vi "HFRR ADV v020 new software.vi"() -> ()   [LabVIEW 2025] (continued)
                    n2485 = Concatenate Strings(w3616, w3615, "Fuel Discription :-" ("Substring"), w3626, w3615, w3636, w3615, "Batch Ref Num :-" ("Substring"), w3612, w3615, " Remarks :- " ("Substring"), w3623, w3615, " Date :- " ("Substring"), w3618, w3615, "Tested By :-" ("Substring"), w3620) -> (w3630:string)
                    "REMARKS" <- w3630
                    n2486 = call <vilib>:"Write Characters To File.vi"("append to file? (new file:F)"=FALSE, "character string"=w3632, "file path (dialog if empty)"=w3600) -> ()  [unwired: 2 in, 1 out]
                    n2487 = call <vilib>:"Write Characters To File.vi"("append to file? (new file:F)"=FALSE, "character string"=w3630, "file path (dialog if empty)"=w3599) -> ()  [unwired: 2 in, 1 out]
                  }
                  frame #2 {
                    n2488 = local write "Cycles elapsed"(0 ("Cycles elapsed")) -> ()
                    n2489 = local write "cyclecount"(0 ("cyclecount")) -> ()
                    n2490 = local write "Save & Continue"(FALSE ("OK")) -> ()
                    n2491 = local write "autostrtflg"(TRUE ("autostrtflg")) -> ()
                    n2492 = local write "Save"(FALSE ("Save")) -> ()
                    n2493 = Get Date/Time In Seconds() -> (seconds since 1Jan1904=w3655:timestamp)
                    n2494 = To Double Precision Float(number=w3655) -> (double precision float=w3654:dbl)
                    n2495 = local write "acq timer"(w3654) -> ()
                    n2496 = One Button Dialog(message="Please ensure sample is mounted properly and machine is ready in all aspects for testing !", button name ("OK")="Ok") -> ()  [unwired: 1 out]
                  }
                  frame #3 {
                    n2497 = stacked-sequence {
                      frame #0 {
                        n2498 = local write "Main Dashboard Buttons"(T1."Dashboard" ("Main Dashboard Buttons")) -> ()
                        n2499 = local write "Main Tab"(T2."Acquire" ("Main Tab")) -> ()
                      }
                      frame #1 {
                        n2500 = local write "EVENT LOG"("" ("EVENT LOG")) -> ()
                      }
                      frame #2 {
                        n2501 = Wait (ms)(milliseconds to wait=u32 50) -> ()  [unwired: 1 out]
                      }
                      frame #3 {
                        n2502 = disable-structure shown="Disabled" {
                          frame Disabled {
                            n2503 = local read "EVENT LOG"() -> (w3667:string)
                            n2504 = call "Event Log.vi"("Content"="Test Details", "EVENT LOG"=w3667) -> ("EVENT LOG"=w3666:string)  [unwired: 8 in, 1 out]
                            n2505 = local write "EVENT LOG"(w3666) -> ()
                          }
                          frame Enabled {
                          }
                        }
                      }
                      frame #4 {
                        n2506 = Wait (ms)(milliseconds to wait=u32 50) -> ()  [unwired: 1 out]
                      }
                      frame #5 {
                        n2507 = local read "FILE"() -> (w3669:string)
                        n2508 = Concatenate Strings("File Name :" ("Content"), w3669) -> (w3670:string)
                        n2509 = local read "EVENT LOG"() -> (w3673:string)
                        n2510 = call "Event Log.vi"("Content"=w3670, "EVENT LOG"=w3673) -> ("EVENT LOG"=w3672:string)  [unwired: 8 in, 1 out]
                        n2511 = local write "EVENT LOG"(w3672) -> ()
                      }
                      frame #6 {
                        n2512 = Wait (ms)(milliseconds to wait=u32 50) -> ()  [unwired: 1 out]
                      }
                      frame #7 {
                        n2513 = local read "Batch Ref Num :"() -> (w3675:string)
                        n2514 = Concatenate Strings("Batch Ref No :" ("Content"), w3675) -> (w3676:string)
                        n2515 = local read "EVENT LOG"() -> (w3679:string)
                        n2516 = call "Event Log.vi"("Content"=w3676, "EVENT LOG"=w3679) -> ("EVENT LOG"=w3678:string)  [unwired: 8 in, 1 out]
                        n2517 = local write "EVENT LOG"(w3678) -> ()
                      }
                      frame #8 {
                        n2518 = Wait (ms)(milliseconds to wait=u32 50) -> ()  [unwired: 1 out]
                      }
                      frame #9 {
                        n2519 = local read "tested by"() -> (w3681:string)
                        n2520 = Concatenate Strings("Tested By :" ("Content"), w3681) -> (w3682:string)
                        n2521 = local read "EVENT LOG"() -> (w3685:string)
                        n2522 = call "Event Log.vi"("Content"=w3682, "EVENT LOG"=w3685) -> ("EVENT LOG"=w3684:string)  [unwired: 8 in, 1 out]
                        n2523 = local write "EVENT LOG"(w3684) -> ()
                      }
                      frame #10 {
                        n2524 = Wait (ms)(milliseconds to wait=u32 50) -> ()  [unwired: 1 out]
                      }
                      frame #11 {
                        n2525 = local read "TEST STANDARD"() -> (w3688:T3)
                        n2526 = case shown="\"ASTM D6079\", Default" w3688 {
                          tunnel: ["ASTM D6079" "ISO 12156" "CEC F-096-A-06" "Custom"] -> w3687
                          frame "ASTM D6079", Default {
                          }
                          frame "ISO 12156" {
                          }
                          frame "CEC F-096-A-06" {
                          }
                          frame "Custom" {
                          }
                        }
                        n2527 = Concatenate Strings("Test Standard :" ("Content"), w3687) -> (w3689:string)
                        n2528 = local read "EVENT LOG"() -> (w3692:string)
                        n2529 = call "Event Log.vi"("Content"=w3689, "EVENT LOG"=w3692) -> ("EVENT LOG"=w3691:string)  [unwired: 8 in, 1 out]
                        n2530 = local write "EVENT LOG"(w3691) -> ()
                      }
                      frame #12 {
                        n2531 = Wait (ms)(milliseconds to wait=u32 50) -> ()  [unwired: 1 out]
                      }
                      frame #13 {
                        n2532 = local read "Fuel Discription :"() -> (w3698:string)
                        n2533 = Concatenate Strings("Fuel Description :" ("Content"), w3698) -> (w3699:string)
                        n2534 = local read "EVENT LOG"() -> (w3702:string)
                        n2535 = call "Event Log.vi"("Content"=w3699, "EVENT LOG"=w3702) -> ("EVENT LOG"=w3701:string)  [unwired: 8 in, 1 out]
                        n2536 = local write "EVENT LOG"(w3701) -> ()
                      }
                      frame #14 {
                        n2537 = Wait (ms)(milliseconds to wait=u32 50) -> ()  [unwired: 1 out]
                      }
                      frame #15 {
                        n2538 = local read "Remarks :"() -> (w3704:string)
                        n2539 = Concatenate Strings("Remarks :" ("Content"), w3704) -> (w3705:string)
                        n2540 = local read "EVENT LOG"() -> (w3708:string)
                        n2541 = call "Event Log.vi"("Content"=w3705, "EVENT LOG"=w3708) -> ("EVENT LOG"=w3707:string)  [unwired: 8 in, 1 out]
                        n2542 = local write "EVENT LOG"(w3707) -> ()
                      }
                      frame #16 {
                        n2543 = Wait (ms)(milliseconds to wait=u32 50) -> ()  [unwired: 1 out]
                      }
                      frame #17 {
                        n2544 = local read "Operator ID"() -> (w3710:string)
                        n2545 = Concatenate Strings("Operator ID :" ("Content"), w3710) -> (w3712:string)
                        n2546 = local read "EVENT LOG"() -> (w3714:string)
                        n2547 = call "Event Log.vi"("Content"=w3712, "EVENT LOG"=w3714) -> ("EVENT LOG"=w3713:string)  [unwired: 8 in, 1 out]
                        n2548 = local write "EVENT LOG"(w3713) -> ()
                      }
                      frame #18 {
                        n2549 = Wait (ms)(milliseconds to wait=u32 50) -> ()  [unwired: 1 out]
                      }
                      frame #19 {
                        n2550 = disable-structure shown="Disabled" {
                          frame Disabled {
                            n2551 = local read "EVENT LOG"() -> (w3718:string)
                            n2552 = call "Event Log.vi"("Content"="Test Parameter", "EVENT LOG"=w3718) -> ("EVENT LOG"=w3717:string)  [unwired: 8 in, 1 out]
                            n2553 = local write "EVENT LOG"(w3717) -> ()
                          }
                          frame Enabled {
                          }
                        }
                      }
                      frame #20 {
                        n2554 = Wait (ms)(milliseconds to wait=u32 50) -> ()  [unwired: 1 out]
                      }
                      frame #21 {
                        n2555 = local read "Set Hz"() -> (w3722:dbl)
                        n2556 = Number To Fractional String(number=w3722, precision (6)=i16 2) -> (F-format string=w3721:string)  [unwired: 2 in]
                        n2557 = Concatenate Strings("Set Frequency [Hz] :" ("Content"), w3721) -> (w3724:string)
                        n2558 = local read "EVENT LOG"() -> (w3726:string)
                        n2559 = call "Event Log.vi"("Content"=w3724, "EVENT LOG"=w3726) -> ("EVENT LOG"=w3725:string)  [unwired: 8 in, 1 out]
                        n2560 = local write "EVENT LOG"(w3725) -> ()
                      }
                      frame #22 {
                        n2561 = Wait (ms)(milliseconds to wait=u32 50) -> ()  [unwired: 1 out]
                      }
                      frame #23 {
                        n2562 = local read "NORMAL LOAD"() -> (w3729:dbl)
                        n2563 = Number To Fractional String(number=w3729, precision (6)=i16 2) -> (F-format string=w3730:string)  [unwired: 2 in]
                        n2564 = Concatenate Strings("Applied Load [grams] :" ("Content"), w3730) -> (w3732:string)
                        n2565 = local read "EVENT LOG"() -> (w3734:string)
                        n2566 = call "Event Log.vi"("Content"=w3732, "EVENT LOG"=w3734) -> ("EVENT LOG"=w3733:string)  [unwired: 8 in, 1 out]
                        n2567 = local write "EVENT LOG"(w3733) -> ()
                      }
                      frame #24 {
                        n2568 = Wait (ms)(milliseconds to wait=u32 50) -> ()  [unwired: 1 out]
                      }
                      frame #25 {
                        n2569 = local read "Set Strk"() -> (w3737:dbl)
                        n2570 = Number To Fractional String(number=w3737, precision (6)=i16 2) -> (F-format string=w3738:string)  [unwired: 2 in]
                        n2571 = Concatenate Strings("Set Stroke [mm] :" ("Content"), w3738) -> (w3740:string)
                        n2572 = local read "EVENT LOG"() -> (w3742:string)
                        n2573 = call "Event Log.vi"("Content"=w3740, "EVENT LOG"=w3742) -> ("EVENT LOG"=w3741:string)  [unwired: 8 in, 1 out]
                        n2574 = local write "EVENT LOG"(w3741) -> ()
                      }
                      frame #26 {
                        n2575 = Wait (ms)(milliseconds to wait=u32 50) -> ()  [unwired: 1 out]
                      }
                      frame #27 {
                        n2576 = local read "Set Temp"() -> (w3745:dbl)
                        n2577 = Number To Fractional String(number=w3745, precision (6)=i16 2) -> (F-format string=w3746:string)  [unwired: 2 in]
                        n2578 = Concatenate Strings("Set Temperature [deg C] :" ("Content"), w3746) -> (w3748:string)
                        n2579 = local read "EVENT LOG"() -> (w3750:string)
                        n2580 = call "Event Log.vi"("Content"=w3748, "EVENT LOG"=w3750) -> ("EVENT LOG"=w3749:string)  [unwired: 8 in, 1 out]
                        n2581 = local write "EVENT LOG"(w3749) -> ()
                      }
                      frame #28 {
                        n2582 = Wait (ms)(milliseconds to wait=u32 50) -> ()  [unwired: 1 out]
                      }
                      frame #29 {
                        n2583 = local read "Set Rh"() -> (w3753:dbl)
                        n2584 = Number To Fractional String(number=w3753, precision (6)=i16 2) -> (F-format string=w3754:string)  [unwired: 2 in]
                        n2585 = Concatenate Strings("Set Humidity [%RH] :" ("Content"), w3754) -> (w3756:string)
                        n2586 = local read "EVENT LOG"() -> (w3758:string)
                        n2587 = call "Event Log.vi"("Content"=w3756, "EVENT LOG"=w3758) -> ("EVENT LOG"=w3757:string)  [unwired: 8 in, 1 out]
                        n2588 = local write "EVENT LOG"(w3757) -> ()
                      }
                      frame #30 {
                        n2589 = Wait (ms)(milliseconds to wait=u32 50) -> ()  [unwired: 1 out]
                      }
                      frame #31 {
                        n2590 = local read "test time"() -> (w3761:dbl)
                        n2591 = Number To Fractional String(number=w3761, precision (6)=i16 1) -> (F-format string=w3762:string)  [unwired: 2 in]
                        n2592 = Concatenate Strings("Test Duration [mins] :" ("Content"), w3762) -> (w3764:string)
                        n2593 = local read "EVENT LOG"() -> (w3766:string)
                        n2594 = call "Event Log.vi"("Content"=w3764, "EVENT LOG"=w3766) -> ("EVENT LOG"=w3765:string)  [unwired: 8 in, 1 out]
                        n2595 = local write "EVENT LOG"(w3765) -> ()
                      }
                      frame #32 {
                        w3767 = dbl[] [] ("History Data")
                        w3768 = cluster{"y":dbl, dbl, "y":dbl}[] [] ("History Data")
                        w3769 = FALSE ("Visible")
                        n2596 = property on="Stroke ( mm )" class="WFChart (strict)"("History Data"=w3768) -> ()  [unwired: 2 in, 2 out]
                        n2597 = property on="Humidity ( %RH )" class="WFChart (strict)"("History Data"=w3767) -> ()  [unwired: 2 in, 2 out]
                        n2598 = property on="Temperature ( Deg C )" class="WFChart (strict)"("History Data"=w3767) -> ()  [unwired: 2 in, 2 out]
                        n2599 = property on="Electrical Contact Resistance ( % )" class="WFChart (strict)"("History Data"=w3767) -> ()  [unwired: 2 in, 2 out]
                        n2600 = property on="Coefficient of Friction" class="WFChart (strict)"("History Data"=w3767) -> ()  [unwired: 2 in, 2 out]
                        n2601 = property on="Frictional Force ( N )" class="WFChart (strict)"("History Data"=w3767) -> ()  [unwired: 2 in, 2 out]
                        n2602 = property on="Coefficient of Friction" class="WFChart (strict)"("History Data"=w3767) -> ()  [unwired: 2 in, 2 out]
                        n2603 = property on="Frictional Force ( N )" class="WFChart (strict)"("History Data"=w3767) -> ()  [unwired: 2 in, 2 out]
                        n2604 = property on="Electrical Contact Resistance ( % )" class="WFChart (strict)"("History Data"=w3767) -> ()  [unwired: 2 in, 2 out]
                        n2605 = property on="Humidity ( %RH )" class="WFChart (strict)"("History Data"=w3767) -> ()  [unwired: 2 in, 2 out]
                        n2606 = property on="Stroke ( mm )" class="WFChart (strict)"("History Data"=w3768) -> ()  [unwired: 2 in, 2 out]
                        n2607 = property on="Temperature ( Deg C )" class="WFChart (strict)"("History Data"=w3767) -> ()  [unwired: 2 in, 2 out]
                        n2608 = property on="Service Password Log" class="Str"("Visible"=w3769) -> ()  [unwired: 2 in, 2 out]
                        n2609 = property on="Password 3" class="Clust (strict)"("Visible"=w3769) -> ()  [unwired: 2 in, 2 out]
                      }
                    }
                    "TEST FILE NAM,E SAVED" <- TRUE ("TEST FILE NAM,E SAVED")
                  }
                }
              }
            }
          }
        }
        n2610 = case shown="True" w3066 {
          frame False {
            n2611 = local write "tfalg"(0.0 ("tfalg")) -> ()
          }
          frame True {
            n2612 = local read "tfalg"() -> (w3211:dbl)
            n2613 = Equal?(x=w3211, y=0.0) -> (x = y?=w3212:bool)
            n2614 = case shown="True" w3212 {
              frame False {
              }
              frame True {
                n2615 = local read "Total No. of Tests"() -> (w3215:dbl)
                n2616 = local write "tfalg"(1.0 ("tfalg")) -> ()
                n2617 = local write "acq 2"(FALSE ("acq 2")) -> ()
                n2618 = Wait (ms)(milliseconds to wait=u32 200) -> ()  [unwired: 1 out]
                n2619 = Increment(x=w3215) -> (x+1=w3214:dbl)
                n2620 = local write "Total No. of Tests"(w3214) -> ()
              }
            }
          }
        }
        n2621 = local write "Test \nStatus"(w3072) -> ()
        n2622 = local write "Save"(w3072) -> ()
        n2623 = local read "Main Tab"() -> (w3029:T2)
        n2624 = case shown="True" w3053 {
          tunnel: [FALSE ("RUN") TRUE ("RUN")] -> w3052
          tunnel: [_ 1] -> w3045
          frame False {
          }
          frame True {
          }
        }
        n2625 = In Range and Coerce(upper limit=w3060, x=w3033, lower limit=w3059) -> (In Range?=w3051:bool)  [unwired: 1 out]
        n2626 = In Range and Coerce(upper limit=w3057, x=w3032, lower limit=w3058) -> (In Range?=w3049:bool)  [unwired: 1 out]
        n2627 = case shown="True" w3065 {
          frame False {
            n2628 = local read "Rt 3"() -> (w3193:bool)
            n2629 = case shown="True" w3193 {
              frame False {
              }
              frame True {
                n2630 = local write "Rt 3"(FALSE ("Rt 3")) -> ()
                n2631 = local write "Json End Flg"(TRUE ("Upld AR 2")) -> ()
              }
            }
            "Rt" <- TRUE ("Rt")
            "Rt 2" <- FALSE ("Rt")
          }
          frame True {
            n2632 = local read "Rt"() -> (w3200:bool)
            n2633 = local write "Rt 2"(TRUE ("Rt 2")) -> ()
            n2634 = case shown="True" w3200 {
              frame False {
              }
              frame True {
                w3201 = TRUE ("Upld AR 2")
                n2635 = local write "Rt"(FALSE ("Rt")) -> ()
                n2636 = local write "Upld AR"(w3201) -> ()
                n2637 = local write "Json St Flg"(w3201) -> ()
              }
            }
            "Rt 3" <- TRUE ("Rt 3")
          }
        }
        n2638 = case shown="True" w3051 {
          tunnel: [FALSE ("RUN") TRUE ("RUN")] -> w3050
          tunnel: [_ 2] -> w3044
          frame False {
          }
          frame True {
          }
        }
        n2639 = case shown="True" w3049 {
          tunnel: [FALSE ("RUN") TRUE ("RUN")] -> w3048
          tunnel: [_ 3] -> w3043
          frame False {
          }
          frame True {
          }
        }
        n2640 = case shown="\"Acquire\"" w3029 {
          tunnel: w3031 -> [_ w3262]
          frame Default {
            w3261 = 0.0 ("output")
            n2641 = local write "PID-out"(w3261) -> ()
            n2642 = local write "Frequency ( Hz )"(w3261) -> ()
          }
          frame "Acquire" {
            n2643 = stacked-sequence {
              frame #0 {
                n2644 = local read "Auto Start Test"() -> (w3264:bool)
                n2645 = case shown="True" w3264 {
                  tunnel: "RUN" -> [w3285 w3288]
                  tunnel: [w3285 w3287] -> w3265
                  frame False {
                  }
                  frame True {
                    n2646 = local read "Auto Start Temp"() -> (w3286:bool)
                    n2647 = Or(x=w3288, y=w3286) -> (x .or. y?=w3287:bool)
                  }
                }
                n2648 = local read "clk"() -> (w3284:dbl)
                n2649 = local read "Save"() -> (w3280:bool)
                n2650 = Equal?(x=w3284, y=0.0) -> (x = y?=w3281:bool)
                n2651 = And(x=w3281, y=w3280) -> (x .and. y?=w3282:bool)
                n2652 = Not(x="Engage") -> (.not. x?=w3271:bool)
                n2653 = case shown="False" w3265 {
                  tunnel: [0.0 w3311] -> w3267
                  frame False {
                    (unwired) TRUE ("Visible")
                    n2654 = local read "Auto Start Test"() -> (w3292:bool)
                    n2655 = local write "Start Time"(TRUE ("Start Time")) -> ()
                    n2656 = property on="Stroke 2" class="DigNum (strict)"("Visible"=FALSE) -> ()  [unwired: 2 in, 2 out]
                    n2657 = case shown="False" w3292 {
                      frame False {
                        n2658 = property on="Heater Button" class="Bool (strict)"("DisabledEnum"=T19."Enabled" ("Disabled")) -> ()  [unwired: 2 in, 2 out]
                        n2659 = property on="Humidity" class="Bool (strict)"("DisabledEnum"=T19."Enabled" ("Disabled")) -> ()  [unwired: 2 in, 2 out]
                      }
                      frame True {
                      }
                    }
                    n2660 = case shown="False" "TestCompFlg" {
                      frame False {
                        n2661 = local read "StartFlg"() -> (w3300:bool)
                        n2662 = case shown="True" w3300 {
                          frame False {
                          }
                          frame True {
                            n2663 = stacked-sequence {
                              frame #0 {
                                n2664 = local read "EVENT LOG"() -> (w3304:string)
                                n2665 = call "Event Log.vi"("Content"="Test was interrupted", "EVENT LOG"=w3304) -> ("EVENT LOG"=w3305:string)  [unwired: 8 in, 1 out]
                                n2666 = local write "EVENT LOG"(w3305) -> ()
                                n2667 = property on="RUN" class="Bool (strict)"("Visible"=TRUE) -> ()  [unwired: 2 in, 2 out]
                                n2668 = property on="Auto Start Test" class="Bool (strict)"("Visible"=TRUE) -> ()  [unwired: 2 in, 2 out]
                              }
                              frame #1 {
                                w3307 = FALSE ("StartFlg")
                                n2669 = property on="Heater Button" class="Bool (strict)"("Val(Sgnl)"=FALSE ("Value (Signaling)")) -> ()  [unwired: 2 in, 2 out]
                                n2670 = local write "Heater Button"(w3307) -> ()
                                n2671 = local write "StartFlg"(w3307) -> ()
                                n2672 = local write "Humidity"(w3307) -> ()
                              }
                              frame #2 {
                                n2673 = local write "Command"("VC;0" ("Command")) -> ()
                              }
                              frame #3 {
                                n2674 = Wait (ms)(milliseconds to wait=u32 1500) -> ()  [unwired: 1 out]
                              }
                              frame #4 {
                                n2675 = local write "Command"("HE;0" ("Command")) -> ()
                              }
                            }
                          }
                        }
                      }
                      frame True {
                      }
                    }
                    n2676 = local write "String 14"("Test will autostart once parameters reach the set value." ("String 14")) -> ()
                  }
                  frame True {
                    (unwired) FALSE ("Visible")
                    n2677 = property on="Stroke 2" class="DigNum (strict)"("Visible"=TRUE) -> ()  [unwired: 2 in, 2 out]
                    n2678 = property on="STOP 2" class="Bool (strict)"("Disabled"=u8 2) -> ()  [unwired: 2 in, 2 out]
                    n2679 = local write "String 14"(" Running....." ("String 14")) -> ()
                    n2680 = property on="Heater Button" class="Bool (strict)"("DisabledEnum"=T19."Disabled and Grayed Out" ("Disabled")) -> ()  [unwired: 2 in, 2 out]
                    n2681 = property on="Humidity" class="Bool (strict)"("DisabledEnum"=T19."Disabled and Grayed Out" ("Disabled")) -> ()  [unwired: 2 in, 2 out]
                    n2682 = case shown="True" "Start Time" {
                      selector: "Start Time" -> [_ w3330]
                      frame False {
                      }
                      frame True {
                        n2683 = Not(x=w3330) -> (.not. x?=w3329:bool)
                        n2684 = local write "Start Time"(w3329) -> ()
                        n2685 = local read "EVENT LOG"() -> (w3331:string)
                        n2686 = call "Event Log.vi"("Content"="Test in progress", "EVENT LOG"=w3331) -> ("EVENT LOG"=w3333:string)  [unwired: 8 in, 1 out]
                        n2687 = local write "EVENT LOG"(w3333) -> ()
                      }
                    }
                    n2688 = disable-structure shown="Enabled" {
                      disable-tunnel: [w3322 w3328] -> w3311
                      frame Disabled {
                        n2689 = local read "Set Hz"() -> (w3325:dbl)
                        n2690 = call <vilib>:"Uniform White Noise Waveform.vi"() -> ("signal out"=w3324:waveform(dbl))  [unwired: 10 in, 1 out]
                        n2691 = Random Number (0-1)() -> (number: 0 to 1=w3321:dbl)
                        n2692 = Add(x=w3325, y=w3324) -> (x+y=w3323:waveform(dbl))
                        n2693 = Multiply(x=ext 0.01 ("y"), y=w3321) -> (x*y=w3319:ext)
                        n2694 = Multiply(x=w3323, y=w3319) -> (x*y=w3322:waveform(ext))
                      }
                      frame Enabled {
                        n2695 = call-poly <vilib>:"Random Number (Range).vi"("lower bound (0)"=49.89, "upper bound (100)"=50.8) -> ("number"=w3328:dbl)  [unwired: 9 in]
                      }
                    }
                    "StartFlg" <- TRUE ("StartFlg")
                  }
                }
                n2696 = case shown="True" w3282 {
                  frame False {
                  }
                  frame True {
                    n2697 = local write "clk"(10.0 ("clk")) -> ()
                    n2698 = Get Date/Time In Seconds() -> (seconds since 1Jan1904=w3336:timestamp)
                    n2699 = To Double Precision Float(number=w3336) -> (double precision float=w3334:dbl)
                    n2700 = local write "acq timer"(w3334) -> ()
                    n2701 = local write "act save time"(w3334) -> ()
                  }
                }
                n2702 = call "Elapsed Time"("Time Target (s)"="Countdown", "Reset"=w3271) -> ("Elapsed Time (s)"=w3276:dbl, "Time has Elapsed"=w3274:bool)  [unwired: 10 in, 6 out]
                "Countdown 2" <- w3276
                n2703 = Subtract(x=w3276, y=2.0) -> (x-y=w3279:dbl)
                n2704 = Less?(x=w3279, y="Countdown") -> (x < y?=w3277:bool)
                n2705 = And(x=w3277, y=w3274) -> (x .and. y?=w3273:bool)
                n2706 = case shown="True" w3273 {
                  frame False {
                  }
                  frame True {
                    (unwired) dbl[] [] ("History Data")
                    n2707 = local write "Engage"(FALSE ("Engage")) -> ()
                    n2708 = local write "RUN"(TRUE ("RUN")) -> ()
                    n2709 = local read "Humidity ( %RH )"() -> (→"Rh Before":dbl)
                  }
                }
                n2710 = local read "Test \nStatus"() -> (w3269:bool)
                n2711 = Select(t=w3267, s=w3269, f=0.0) -> (s? t:f=w3268:dbl)
                n2712 = local write "Frequency ( Hz )"(w3268) -> ()
              }
              frame #1 {
                w3359 = 1000000.0 ("x")
                # "HC;1/0\nST;VALUE"
                # "Elapsed time\ncof\nstroke\nAir temp\nTemp\nHumidity"
                # "acq timer\n\nact save time"
                # "convert to microseconds"
                n2713 = local read "COUNT"() -> (w3342:i32)
                n2714 = local read "Rate"() -> (w3355:dbl)
                n2715 = Divide(x=w3359, y=w3355) -> (x/y=w3360:dbl)
                n2716 = Greater Or Equal?(x=w3342, y=250) -> (x >= y?=w3341:bool)
                n2717 = Get Date/Time In Seconds() -> (seconds since 1Jan1904=w3362:timestamp)
                n2718 = case shown="True" w3341 {
                  frame False {
                    n2719 = local read "COUNT"() -> (w3363:i32)
                    n2720 = Increment(x=w3363) -> (x+1=w3364:i32)
                    n2721 = local write "COUNT"(w3364) -> ()
                  }
                  frame True {
                    n2722 = local write "COUNT"(0 ("COUNT")) -> ()
                  }
                }
                n2723 = local read "Samplingtime 2"() -> (w3340:dbl)
                n2724 = local read "act save time"() -> (w3357:dbl)
                n2725 = Divide(x=w3360, y=w3359) -> (x/y=w3358:dbl)
                n2726 = To Double Precision Float(number=w3362) -> (double precision float=w3351:dbl)
                n2727 = Add(x=w3357, y=w3340) -> (x+y=w3356:dbl)
                n2728 = local read "acq timer"() -> (w3361:dbl)
                n2729 = local read "COUNT"() -> (w3344:i32)
                n2730 = Greater Or Equal?(x=w3351, y=w3356) -> (x >= y?=w3339:bool)
                n2731 = Multiply(x=w3358, y=w3344) -> (x*y=w3350:dbl)
                n2732 = Subtract(x=w3351, y=w3361) -> (x-y=w3353:dbl)
                n2733 = local read "Save"() -> (w3354:bool)
                n2734 = Add(x=w3353, y=w3350) -> (x+y=w3337:dbl)
                "Elapsed time 3" <- w3337
                n2735 = And(x=w3339, y=w3354) -> (x .and. y?=w3352:bool)
                n2736 = Divide(x=w3337, y=60.0) -> (x/y=w3348:dbl)
                n2737 = local read "Test \nStatus"() -> (w3338:bool)
                n2738 = local read "clk"() -> (w3345:dbl)
                n2739 = Equal?(x=w3345, y=10.0) -> (x = y?=w3347:bool)
                n2740 = case shown="True" w3352 {
                  tunnel: w3351 -> [_ w3475]
                  tunnel: [FALSE ("Boolean 2") TRUE ("Boolean 2")] -> _
                  frame False {
                  }
                  frame True {
                    w3429 = ";" ("Substring")
                    # "Pid out/\nFreq response value"
                    n2741 = local write "act save time"(w3475) -> ()
                    n2742 = local read "FILE"() -> (w3423:string)
                    n2743 = call "file check.vi"("file name in"=w3423) -> ("error out"=w3426:errorcluster, "file name out"=w3421:string)  [unwired: 9 in]
                    n2744 = local read "LVDT STROKE"() -> (w3418:dbl)
                    n2745 = local read "Add up Stroke"() -> (w3416:dbl)
                    n2746 = call "FILE PATH CREATION.vi"("error in"=w3426, "FILE NAME :"=w3421) -> ("FILE OUT"=w3424:path)  [unwired: 8 in, 1 out]
                    n2747 = Concatenate Strings(w3421, ".dgf" ("Substring")) -> (w3425:string)
                    n2748 = Subtract(x=w3418, y=w3416) -> (x-y=w3417:dbl)
                    n2749 = Absolute Value(x=w3417) -> (abs(x)=w3415:dbl)
                    n2750 = local read "FF 2"() -> (→"Frictional Force ( N )" →"Frictional Force ( N )":dbl)
                    n2751 = Build Path(base path=w3424, name or relative path=w3425) -> (appended path=w3420:path)
                    n2752 = local read "COF 2"() -> (w3434:dbl)
                    "cof" <- w3434
                    "Coefficient of Friction" <- w3434
                    "COF 4" <- w3434
                    "Coefficient of Friction" <- w3434
                    n2753 = local read "TEMP"() -> (w3437:dbl)
                    "Temp" <- w3437
                    "Temperature ( Deg C )" <- w3437
                    n2754 = local read "Humidity ( %RH )"() -> (w3436:dbl)
                    "Humidity ( %RH )" <- w3436
                    "Humidity ( %RH )" <- w3436
                    n2755 = local read "Frequency ( Hz )"() -> (w3443:dbl)
                    n2756 = call <vilib>:"Mean PtByPt.vi"("x"=w3415, "sample length"="STROKE FILTER") -> ("mean"=w3414:dbl)  [unwired: 2 in, 1 out]
                    n2757 = local read "Elapsed time"() -> (w3468:dbl)
                    n2758 = local read "AIR TEMP"() -> (w3441:dbl)
                    n2759 = local read "PID-out"() -> (w3446:dbl)
                    n2760 = local write "Temperature ( Deg C )"(w3437) -> ()
                    n2761 = Number To Fractional String(number=w3414, width (-)=i16 9 ("precision (6)"), precision (6)=i16 6) -> (F-format string=w3461:string)  [unwired: 1 in]
                    n2762 = Number To Fractional String(number=w3441, width (-)=i16 9 ("precision (6)"), precision (6)=i16 3) -> (F-format string=w3460:string)  [unwired: 1 in]
                    n2763 = Number To Fractional String(number=w3437, width (-)=i16 9 ("precision (6)"), precision (6)=i16 3) -> (F-format string=w3457:string)  [unwired: 1 in]
                    n2764 = Number To Fractional String(number=w3436, width (-)=i16 9 ("precision (6)"), precision (6)=i16 3) -> (F-format string=w3454:string)  [unwired: 1 in]
                    n2765 = Number To Fractional String(number=0.0, width (-)=i16 9 ("precision (6)"), precision (6)=i16 3) -> (F-format string=w3451:string)  [unwired: 1 in]
                    n2766 = Number To Fractional String(number=w3446, width (-)=i16 9 ("precision (6)"), precision (6)=i16 3) -> (F-format string=w3447:string)  [unwired: 1 in]
                    n2767 = Number To Fractional String(number=w3443, width (-)=i16 9 ("precision (6)"), precision (6)=i16 3) -> (F-format string=w3442:string)  [unwired: 1 in]
                    n2768 = Number To Fractional String(number=w3434, width (-)=i16 9 ("precision (6)"), precision (6)=i16 6) -> (F-format string=w3469:string)  [unwired: 1 in]
                    n2769 = Number To Fractional String(number=w3468, width (-)=i16 14 ("precision (6)"), precision (6)=i16 3) -> (F-format string=w3470:string)  [unwired: 1 in]
                    n2770 = Bundle("y"=1.02, "mean"=w3414, "y"=0.98) -> (w3435:cluster{"y":dbl, "mean":dbl, "y":dbl})  [unwired: 1 in]
                    n2771 = Number To Fractional String(number="Ambient Humidity :", width (-)=i16 9 ("precision (6)"), precision (6)=i16 6) -> (F-format string=w3427:string)  [unwired: 1 in]
                    n2772 = local read "RUN"() -> (w3433:bool)
                    n2773 = case shown="True" w3433 {
                      tunnel: w3435 -> [_ w3480]
                      tunnel: w3414 -> [_ w3479]
                      tunnel: w3414 -> [_ w3477]
                      tunnel: w3414 -> [_ w3478]
                      frame False {
                      }
                      frame True {
                        "Stroke ( mm )" <- w3480
                        "Stroke ( mm )" <- w3480
                        "Stroke 4" <- w3479
                        "Stroke 3" <- w3477
                        "Stroke 2" <- w3478
                        "measured_stroke" <- w3477
                      }
                    }
                    n2774 = Concatenate Strings(w3470, w3429, w3469, w3429, w3461, w3429, w3460, w3429, w3457, w3429, w3454, w3429, w3451, w3429, w3447, w3429, w3442, w3429, w3427, "\r") -> (w3467:string)
                    n2775 = call <vilib>:"Write Characters To File.vi"("append to file? (new file:F)"=TRUE, "character string"=w3467, "file path (dialog if empty)"=w3420) -> ()  [unwired: 2 in, 1 out]
                    "refresh flag" <- TRUE ("refresh flag")
                  }
                }
                n2776 = case shown="True" w3338 {
                  tunnel: w3348 -> [_ w3374]
                  tunnel: w3353 -> [_ w3384]
                  tunnel: [0.0 w3380] -> _
                  tunnel: w3347 -> [_ w3379]
                  tunnel: [0.0 w3378] -> _
                  tunnel: w3337 -> [_ w3378]
                  tunnel: w3351 -> [w3367 _]
                  frame False {
                    n2777 = local write "acq timer"(w3367) -> ()
                    n2778 = local write "Test Duration Status"(0.0 ("Test Duration Status")) -> ()
                  }
                  frame True {
                    n2779 = local read "Set Hz"() -> (w3381:dbl)
                    n2780 = local write "Elapsed time"(w3374) -> ()
                    n2781 = local read "test time"() -> (w3373:dbl)
                    n2782 = Multiply(x=w3384, y=w3381) -> (x*y=w3383:dbl)
                    n2783 = case shown="False" w3379 {
                      tunnel: w3383 -> [w3385 _]
                      tunnel: [w3385 1.0] -> w3380
                      frame False {
                        n2784 = local write "Cycles elapsed"(w3385) -> ()
                      }
                      frame True {
                      }
                    }
                    n2785 = Greater?(x=w3374, y=w3373) -> (0:w3382:bool)
                    n2786 = Subtract(x=w3373, y=w3374) -> (x-y=w3372:dbl)
                    "time" <- w3372
                    n2787 = Multiply(x=w3372, y=60.0) -> (x*y=w3371:dbl)
                    n2788 = local write "Time Remaining"(w3371) -> ()
                    n2789 = local write "Remaining Time"(w3371) -> ()
                    n2790 = case shown="True" w3382 {
                      frame False {
                      }
                      frame True {
                        n2791 = stacked-sequence {
                          frame #0 {
                            w3390 = T19."Enabled" ("Disabled")
                            w3389 = FALSE ("TEST FILE NAM,E SAVED")
                            w3391 = "" ("FILE")
                            w3392 = TRUE ("Visible")
                            n2792 = local write "Humidity"(FALSE ("Humidity")) -> ()
                            n2793 = local write "RUN"(FALSE ("OK Button 2")) -> ()
                            n2794 = local write "Heater Button"(FALSE ("Heater Button")) -> ()
                            n2795 = local write "Auto Start Test"(FALSE ("Auto Start Test")) -> ()
                            n2796 = local write "TestCompFlg"(TRUE ("StpFlg")) -> ()
                            n2797 = local read "Humidity ( %RH )"() -> (→"Rh After":dbl)
                            n2798 = property on="STOP 2" class="Bool (strict)"("Disabled"=u8 0) -> ()  [unwired: 2 in, 2 out]
                            n2799 = local read "EVENT LOG"() -> (w3397:string)
                            n2800 = call "Event Log.vi"("Content"="Test Completed", "EVENT LOG"=w3397) -> ("EVENT LOG"=w3396:string)  [unwired: 8 in, 1 out]
                            n2801 = property on="RUN" class="Bool (strict)"("Visible"=w3392) -> ()  [unwired: 2 in, 2 out]
                            n2802 = property on="Auto Start Test" class="Bool (strict)"("Visible"=w3392) -> ()  [unwired: 2 in, 2 out]
                            n2803 = local write "Batch Ref Num :"(w3391) -> ()
                            n2804 = local write "FILE"(w3391) -> ()
                            n2805 = local write "EVENT LOG"(w3396) -> ()
                            n2806 = local write "TEST FILE NAM,E SAVED"(w3389) -> ()
                            n2807 = local write "Fuel Discription :"(w3391) -> ()
                            n2808 = local write "START TEMP"(w3389) -> ()
                            n2809 = local write "Remarks :"(w3391) -> ()
                            n2810 = local write "Main Dashboard Buttons"(T1."Imaging" ("Main Dashboard Buttons")) -> ()
                            n2811 = local write "Main Tab"(T2."Adv Scar" ("Main Tab")) -> ()
                            n2812 = property on="FRICVALZ 2" class="Bool (strict)"("DisabledEnum"=w3390) -> ()  [unwired: 2 in, 2 out]
                            n2813 = property on="FRICVALZ 3" class="Bool (strict)"("DisabledEnum"=w3390) -> ()  [unwired: 2 in, 2 out]
                            n2814 = property on="FRICVALZ 4" class="Bool (strict)"("DisabledEnum"=w3390) -> ()  [unwired: 2 in, 2 out]
                          }
                          frame #1 {
                            n2815 = Wait (ms)(milliseconds to wait=u32 1500) -> ()  [unwired: 1 out]
                          }
                          frame #2 {
                            n2816 = local write "Command"("VC;0") -> ()
                          }
                          frame #3 {
                            n2817 = Wait (ms)(milliseconds to wait=u32 1500) -> ()  [unwired: 1 out]
                          }
                          frame #4 {
                            n2818 = local write "Command"("VC;0") -> ()
                          }
                          frame #5 {
                            n2819 = Wait (ms)(milliseconds to wait=u32 1500) -> ()  [unwired: 1 out]
                          }
                          frame #6 {
                            n2820 = local write "Command"("ST;0") -> ()
                          }
                          frame #7 {
                            n2821 = local write "measured_stroke"(0.0 ("measured_stroke")) -> ()
                            n2822 = Wait (ms)(milliseconds to wait=u32 1500) -> ()  [unwired: 1 out]
                          }
                          frame #8 {
                            n2823 = local write "Command"("HE;0") -> ()
                          }
                        }
                      }
                    }
                    n2824 = Divide(x=w3374, y=w3373) -> (x/y=w3377:dbl)
                    n2825 = Multiply(x=w3377, y=100.0) -> (x*y=w3375:dbl)
                    n2826 = local write "Test Duration Status"(w3375) -> ()
                  }
                }
              }
              frame #2 {
                n2827 = case shown="True" "Heater Button" {
                  tunnel: [0.0 ("output") w3503] -> w3481
                  frame False {
                    w3484 = TRUE ("tmpchk")
                    n2828 = local read "TEMP"() -> (w3485:dbl)
                    n2829 = local write "Temp ini"(w3485) -> ()
                    n2830 = local write "Reset 4"(w3484) -> ()
                    n2831 = local write "tmpchk"(w3484) -> ()
                    n2832 = local write "reinit"(TRUE ("reinit")) -> ()
                    n2833 = local write "manual temp log"(TRUE ("manual temp log")) -> ()
                  }
                  frame True {
                    # "Logic to turn off\nthe heater when \ntemp is not rising.\nTime - 60 sec\nDelta t- 5°c"
                    n2834 = local read "Temp ini"() -> (w3492:dbl)
                    n2835 = local read "Auto Start Test"() -> (w3488:bool)
                    n2836 = Less?(x=w3492, y=53.0) -> (x < y?=w3490:bool)
                    n2837 = case shown="False" w3488 {
                      frame False {
                        n2838 = local read "Set Temp"() -> (w3512:dbl)
                        n2839 = local read "TEMP"() -> (w3511:dbl)
                        n2840 = Subtract(x=w3512, y=w3511) -> (x-y=w3510:dbl)
                        n2841 = Absolute Value(x=w3510) -> (abs(x)=w3509:dbl)
                        n2842 = Less?(x=w3509, y=0.5) -> (x < y?=w3507:bool)
                        n2843 = case shown="True" w3507 {
                          tunnel: "manual temp log" -> [_ w3513]
                          frame False {
                          }
                          frame True {
                            n2844 = case shown="True" w3513 {
                              selector: w3513 -> [_ w3514]
                              frame False {
                              }
                              frame True {
                                # "#Event log"
                                n2845 = Not(x=w3514) -> (.not. x?=w3515:bool)
                                n2846 = local write "manual temp log"(w3515) -> ()
                                n2847 = local read "EVENT LOG"() -> (w3518:string)
                                n2848 = call "Event Log.vi"("Content"="Target Temperature reached", "EVENT LOG"=w3518) -> ("EVENT LOG"=w3517:string)  [unwired: 8 in, 1 out]
                                n2849 = local write "EVENT LOG"(w3517) -> ()
                              }
                            }
                          }
                        }
                      }
                      frame True {
                        n2850 = local write "manual temp log"(TRUE ("manual temp log")) -> ()
                      }
                    }
                    n2851 = And(x="tmpchk", y=w3490) -> (x .and. y?=w3493:bool)
                    n2852 = case shown="True" w3493 {
                      frame False {
                      }
                      frame True {
                        n2853 = call "Elapsed Time8"("Time Target (s)"=300.0, "Reset"="Reset 4") -> ("Time has Elapsed"=w3520:bool)  [unwired: 10 in, 7 out]
                        n2854 = flat-sequence {
                          tunnel: w3520 -> [_]
                          frame #0 {
                            n2855 = local write "Reset 4"(FALSE ("Reset 4")) -> ()
                          }
                        }
                        n2856 = case shown="True" w3520 {
                          frame False {
                          }
                          frame True {
                            n2857 = local read "Temp ini"() -> (w3527:dbl)
                            n2858 = Add(x=w3527, y=5.0) -> (x+y=w3525:dbl)
                            n2859 = local read "TEMP"() -> (w3528:dbl)
                            n2860 = Greater?(x=w3528, y=w3525) -> (0:w3526:bool)
                            n2861 = case shown="False" w3526 {
                              frame False {
                                n2862 = local write "Heater Button"(FALSE ("Heater Button")) -> ()
                              }
                              frame True {
                                n2863 = local write "tmpchk"(FALSE ("tmpchk")) -> ()
                              }
                            }
                          }
                        }
                      }
                    }
                    n2864 = local read "Set Temp"() -> (w3501:dbl)
                    n2865 = local read "TEMP"() -> (w3495:dbl)
                    n2866 = call-poly <vilib>:"PID.vi"("reinitialize? (F)"="reinit", "dt (s)"=-1.0, "process variable"=w3495, "setpoint"=w3501) -> ("output"=w3498:dbl)  [unwired: 6 in, 1 out]
                    n2867 = Subtract(x=w3501, y=w3495) -> (x-y=w3502:dbl)
                    n2868 = Add(x=w3501, y=0.5) -> (x+y=w3499:dbl)
                    n2869 = Greater Or Equal?(x=w3495, y=w3499) -> ()  [unwired: 1 out]
                    n2870 = Select(t=0.0, s=FALSE, f=w3498) -> (s? t:f=w3497:dbl)
                    "PID output" <- w3497
                    n2871 = flat-sequence {
                      tunnel: w3497 -> [w3531]
                      tunnel: [w3531] -> w3503
                      frame #0 {
                        n2872 = local write "reinit"(FALSE ("reinit")) -> ()
                      }
                    }
                    n2873 = Bundle(w3502, "output"=w3497, "TEMP"=w3495) -> ()  [unwired: 1 in, 1 out]
                  }
                }
                "PID-out" <- w3481
              }
              frame #3 {
                n2874 = local read "TEMP"() -> (w3533:dbl)
                n2875 = Greater Or Equal?(x=w3533, y="Set Temp 2") -> (x >= y?=w3538:bool)
                n2876 = case shown="True" w3538 {
                  tunnel: [FALSE TRUE] -> w3536
                  frame False {
                  }
                  frame True {
                  }
                }
                "Status 13" <- w3536
                n2877 = And(x=w3536, y="trip1 8") -> (x .and. y?=w3535:bool)
                n2878 = case shown="True" w3535 {
                  frame False {
                    n2879 = local write "Heater Trip Temp"(TRUE ("Heater Trip Temp")) -> ()
                  }
                  frame True {
                    w3541 = FALSE ("OK Button 2")
                    n2880 = case shown="True" "Heater Trip Temp" {
                      selector: "Heater Trip Temp" -> [_ w3543]
                      frame False {
                      }
                      frame True {
                        n2881 = Not(x=w3543) -> (.not. x?=w3542:bool)
                        n2882 = local read "EVENT LOG"() -> (w3546:string)
                        n2883 = local write "Heater Trip Temp"(w3542) -> ()
                        n2884 = call "Event Log.vi"("Content"="Heater Trip", "EVENT LOG"=w3546) -> ("EVENT LOG"=w3545:string)  [unwired: 8 in, 1 out]
                        n2885 = local write "EVENT LOG"(w3545) -> ()
                      }
                    }
                    n2886 = local write "RUN"(w3541) -> ()
                    n2887 = property on="Auto Start Test" class="Bool (strict)"("Value"=w3541) -> ()  [unwired: 2 in, 2 out]
                    n2888 = local write "Heater Button"(w3541) -> ()
                  }
                }
              }
            }
            n2889 = case shown="False" w3262 {
              frame False {
                n2890 = disable-structure shown="Disabled" {
                  frame Disabled {
                    n2891 = stacked-sequence {
                      frame #0 {
                        n2892 = local write "RUN"(FALSE ("OK Button 2")) -> ()
                      }
                      frame #1 {
                      }
                    }
                  }
                  frame Enabled {
                  }
                }
              }
              frame True {
              }
            }
          }
        }
        n2893 = local read "airtempflg"() -> (w3054:bool)
        n2894 = Or(x=w3054, y=w3052) -> (x .or. y?=w3055:bool)
        n2895 = Insert Into Array(array=string[] ["Air Temperature has reached set value,", "Humidity has reached set value,", "Sample Temperaturehas reached set value,", ""], index=0, new element="") -> (w3040:string[])
        n2896 = Build Array(w3045, w3044, w3043) -> (w3041:i32[])
        n2897 = disable-structure shown="Disabled" {
          disable-tunnel: w3055 -> [w3132 _]
          disable-tunnel: w3050 -> [w3131 _]
          disable-tunnel: w3048 -> [w3130 _]
          frame Disabled {
            n2898 = Compound Arithmetic op=AND(w3132, w3131, w3130) -> ()  [unwired: 1 out]
            n2899 = case shown="True" {
              selector: _ -> [_ _]
              frame False {
              }
              frame True {
                w3133 = FALSE ("autostrtflg")
                n2900 = local write "RUN"(TRUE ("RUN")) -> ()
                n2901 = local write "autostrtflg"(w3133) -> ()
                n2902 = local write "autostart"(w3133) -> ()
                n2903 = local write "String 14"(" Running....." ("String 14")) -> ()
              }
            }
          }
          frame Enabled {
          }
        }
        n2904 = for {
          tunnel: w3041 -> [w3183] mode=indexing
          tunnel: w3040 -> [w3182]
          shift-right: [w3179] -> w3039
          shift-left: "" -> [w3181]
          n2905 = Index Array(array=w3182, index=w3183) -> (element=w3180:string)
          n2906 = Concatenate Strings(w3180, w3181) -> (w3179:string)
        }
        n2907 = local write "autostart 2"(w3039) -> ()
        n2908 = local read "Reset Graph"() -> (w3028:bool)
        n2909 = case shown="True" w3028 {
          selector: w3028 -> [_ w3082]
          frame False {
          }
          frame True {
            w3096 = 0.0 ("X Scale.Range:Maximum")
            n2910 = Not(x=w3082) -> (.not. x?=w3081:bool)
            n2911 = local write "Reset Graph"(w3081) -> ()
            n2912 = property on="Electrical Contact Resistance ( % )" class="WFChart (strict)"("XScale.Maximum"=600.0 ("X Scale.Range:Maximum"), "XScale.Minimum"=0.0 ("X Scale.Range:Minimum"), "YScale.Maximum"=100.0 ("Y Scale.Range:Maximum"), "YScale.Minimum"=0.0 ("Y Scale.Range:Minimum")) -> ()  [unwired: 2 in, 2 out]
            n2913 = property on="Frictional Force ( N )" class="WFChart (strict)"("XScale.Maximum"=600.0 ("X Scale.Range:Maximum"), "XScale.Minimum"=0.0 ("X Scale.Range:Minimum"), "YScale.Maximum"=100.0 ("Y Scale.Range:Maximum"), "YScale.Minimum"=0.0 ("Y Scale.Range:Minimum")) -> ()  [unwired: 2 in, 2 out]
            n2914 = property on="Temperature ( Deg C )" class="WFChart (strict)"("XScale.Maximum"=600.0 ("X Scale.Range:Maximum"), "XScale.Minimum"=0.0 ("X Scale.Range:Minimum"), "YScale.Maximum"=100.0 ("Y Scale.Range:Maximum"), "YScale.Minimum"=0.0 ("Y Scale.Range:Minimum")) -> ()  [unwired: 2 in, 2 out]
            n2915 = property on="Humidity ( %RH )" class="WFChart (strict)"("XScale.Maximum"=600.0 ("X Scale.Range:Maximum"), "XScale.Minimum"=0.0 ("X Scale.Range:Minimum"), "YScale.Maximum"=100.0 ("Y Scale.Range:Maximum"), "YScale.Minimum"=0.0 ("Y Scale.Range:Minimum")) -> ()  [unwired: 2 in, 2 out]
            n2916 = property on="Stroke ( mm )" class="WFChart (strict)"("XScale.Maximum"=600.0 ("X Scale.Range:Maximum"), "XScale.Minimum"=0.0 ("X Scale.Range:Minimum"), "YScale.Maximum"=100.0 ("Y Scale.Range:Maximum"), "YScale.Minimum"=0.0 ("Y Scale.Range:Minimum")) -> ()  [unwired: 2 in, 2 out]
            n2917 = property on="Coefficient of Friction" class="WFChart (strict)"("XScale.Maximum"=600.0 ("X Scale.Range:Maximum"), "XScale.Minimum"=0.0 ("X Scale.Range:Minimum"), "YScale.Maximum"=100.0 ("Y Scale.Range:Maximum"), "YScale.Minimum"=0.0 ("Y Scale.Range:Minimum")) -> ()  [unwired: 2 in, 2 out]
            n2918 = property on="Electrical Contact Resistance ( % )" class="WFChart (strict)"("XScale.Minimum"=0.0 ("X Scale.Range:Minimum"), "XScale.Maximum"=600.0 ("X Scale.Range:Maximum"), "YScale.Minimum"=0.0 ("Y Scale.Range:Minimum"), "YScale.Maximum"=100.0 ("Y Scale.Range:Maximum")) -> ()  [unwired: 2 in, 2 out]
            n2919 = property on="Temperature ( Deg C )" class="WFChart (strict)"("XScale.Minimum"=0.0 ("X Scale.Range:Minimum"), "XScale.Maximum"=600.0 ("X Scale.Range:Maximum"), "YScale.Minimum"=0.0 ("Y Scale.Range:Minimum"), "YScale.Maximum"=100.0 ("Y Scale.Range:Maximum")) -> ()  [unwired: 2 in, 2 out]
            n2920 = property on="Coefficient of Friction" class="WFChart (strict)"("XScale.Minimum"=0.0 ("X Scale.Range:Minimum"), "XScale.Maximum"=600.0 ("X Scale.Range:Maximum"), "YScale.Maximum"=1.0 ("X Scale.Range:Minimum"), "YScale.Minimum"=0.0 ("X Scale.Range:Minimum")) -> ()  [unwired: 2 in, 2 out]
            n2921 = property on="Frictional Force ( N )" class="WFChart (strict)"("XScale.Maximum"=600.0 ("X Scale.Range:Maximum"), "XScale.Minimum"=w3096, "YScale.Maximum"=10.0 ("Y Scale.Range:Maximum"), "YScale.Minimum"=w3096) -> ()  [unwired: 2 in, 2 out]
            n2922 = property on="Stroke ( mm )" class="WFChart (strict)"("XScale.Maximum"=600.0 ("X Scale.Range:Maximum"), "XScale.Minimum"=0.0 ("X Scale.Range:Minimum"), "YScale.Maximum"=100.0 ("Y Scale.Range:Maximum"), "YScale.Minimum"=0.0 ("Y Scale.Range:Minimum")) -> ()  [unwired: 2 in, 2 out]
            n2923 = property on="Humidity ( %RH )" class="WFChart (strict)"("XScale.Maximum"=600.0 ("X Scale.Range:Maximum"), "XScale.Minimum"=0.0 ("X Scale.Range:Minimum"), "YScale.Maximum"=100.0 ("Y Scale.Range:Maximum"), "YScale.Minimum"=0.0 ("Y Scale.Range:Minimum")) -> ()  [unwired: 2 in, 2 out]
          }
        }
      }
      frame "Compare Files" {
        # "Elapsed time\ncof\nstroke\nAir temp\nTemp\nHumidity"
        n2924 = case shown="True" "RSTV1 2" {
          frame False {
          }
          frame True {
            n2925 = property on="Humidity ( %RH )" class="XYGraph (strict)"("Y Scale.Display Format:Precision"=u8 0 ("Y Scale.Format & Precision:Precision")) -> ()  [unwired: 2 in, 2 out]
            n2926 = property on="Humidity ( %RH )" class="XYGraph (strict)"("X Scale.Range:Minimum"=0.0, "X Scale.Range:Maximum"=75.0, "Y Scale.Range:Minimum"=48.0, "Y Scale.Range:Maximum"=58.0) -> ()  [unwired: 2 in, 2 out]
          }
        }
        n2927 = case shown="True" "RST CP 2" {
          frame False {
          }
          frame True {
            n2928 = property on="XY Graph 13" class="XYGraph (strict)"("Y Scale.Display Format:Precision"=u8 0 ("Y Scale.Format & Precision:Precision")) -> ()  [unwired: 2 in, 2 out]
            n2929 = property on="XY Graph 13" class="XYGraph (strict)"("X Scale.Range:Minimum"=0.0, "X Scale.Range:Maximum"=75.0, "Y Scale.Range:Minimum"=0.0, "Y Scale.Range:Maximum"=100.0) -> ()  [unwired: 2 in, 2 out]
          }
        }
        n2930 = case shown="True" "RST CP" {
          frame False {
          }
          frame True {
            n2931 = property on="Sample Temperature ( °C )" class="XYGraph (strict)"("Y Scale.Display Format:Precision"=u8 2 ("Y Scale.Format & Precision:Precision")) -> ()  [unwired: 2 in, 2 out]
            n2932 = property on="Sample Temperature ( °C )" class="XYGraph (strict)"("X Scale.Range:Minimum"=0.0, "X Scale.Range:Maximum"=75.0, "Y Scale.Range:Minimum"=58.0, "Y Scale.Range:Maximum"=62.0) -> ()  [unwired: 2 in, 2 out]
          }
        }
        n2933 = case shown="True" "RSTV1 3" {
          frame False {
          }
          frame True {
            n2934 = property on="Air Temperature  ( °C )" class="XYGraph (strict)"("Y Scale.Display Format:Precision"=u8 2 ("Y Scale.Format & Precision:Precision")) -> ()  [unwired: 2 in, 2 out]
            n2935 = property on="Air Temperature  ( °C )" class="XYGraph (strict)"("X Scale.Range:Minimum"=0.0 ("Y Scale.Range:Minimum"), "X Scale.Range:Maximum"=75.0 ("Y Scale.Range:Maximum"), "Y Scale.Range:Minimum"=20.0 ("X Scale.Range:Minimum"), "Y Scale.Range:Maximum"=26.0 ("X Scale.Range:Maximum")) -> ()  [unwired: 2 in, 2 out]
          }
        }
        n2936 = case shown="True" "RSTV1 4" {
          frame False {
          }
          frame True {
            n2937 = property on="Stroke ( mm )" class="XYGraph (strict)"("Y Scale.Display Format:Precision"=u8 2 ("Y Scale.Format & Precision:Precision")) -> ()  [unwired: 2 in, 2 out]
            n2938 = property on="Stroke ( mm )" class="XYGraph (strict)"("X Scale.Range:Minimum"=0.0 ("Y Scale.Range:Maximum"), "X Scale.Range:Maximum"=75.0 ("X Scale.Range:Minimum"), "Y Scale.Range:Minimum"=0.98, "Y Scale.Range:Maximum"=1.02) -> ()  [unwired: 2 in, 2 out]
          }
        }
        n2939 = case shown="True" "rstv2" {
          frame False {
          }
          frame True {
            n2940 = property on="Coefficient Of Friction" class="XYGraph (strict)"("Y Scale.Display Format:Precision"=u8 3 ("Y Scale.Format & Precision:Precision")) -> ()  [unwired: 2 in, 2 out]
            n2941 = property on="Coefficient Of Friction" class="XYGraph (strict)"("X Scale.Range:Minimum"=0.0 ("Y Scale.Range:Maximum"), "X Scale.Range:Maximum"=75.0, "Y Scale.Range:Minimum"=0.0, "Y Scale.Range:Maximum"=1.0 ("X Scale.Range:Minimum")) -> ()  [unwired: 2 in, 2 out]
          }
        }
        n2942 = case shown="True" "RST CP 3" {
          frame False {
          }
          frame True {
            n2943 = property on="Air Temp ( °C ) vs Humidity ( % RH )" class="XYGraph (strict)"("X Scale.Range:Minimum"=18.0, "X Scale.Range:Maximum"=28.0 ("X Scale.Range:Minimum"), "Y Scale.Range:Minimum"=30.0 ("X Scale.Range:Minimum"), "Y Scale.Range:Maximum"=70.0 ("X Scale.Range:Minimum")) -> ()  [unwired: 2 in, 2 out]
          }
        }
        n2944 = case shown="True" "OPEN 1" {
          frame False {
          }
          frame True {
            (unwired) 0  # existing file
            w3822 = "Choose a datalog file to open"  # prompt
            n2945 = local write "OPEN 1"(FALSE ("OPEN 1")) -> ()
            n2946 = String To Path(string="C:\\LAB-IQ\\Data\\") -> (path=w3807:path)
            n2947 = File Dialog(6:"*.dgf" ("pattern"), 7:w3822, 11:w3807) -> (0:w3805:errorcluster, 3:w3813:path)  [unwired: 4 in, 2 out]
            n2948 = Unbundle(w3805) -> ()  [unwired: 3 out]
            n2949 = Strip Path(path=w3813) -> (name=w3812:string)  [unwired: 1 out]
            n2950 = Path To String(path=w3813) -> (string=w3808:string)
            "string1" <- w3808
            n2951 = Match Pattern(string=w3812, regular expression=".dgf") -> (before substring=→"String Control":string)  [unwired: 1 in, 3 out]
            n2952 = Match Pattern(string=w3808, regular expression=".dgf" ("substring (\"\")")) -> (before substring=w3818:string)  [unwired: 1 in, 3 out]
            n2953 = Concatenate Strings(w3818, ".duf" ("Substring")) -> (w3814:string)
            n2954 = String To Path(string=w3814) -> (path=w3819:path)
            n2955 = call <vilib>:"Read Characters From File.vi"("file path (dialog if empty)"=w3819, "start of read offset (chars.:0)"=60 ("start of read offset (chars.: 0)")) -> ("character string"=→"String Control 2":string)  [unwired: 4 in, 3 out]
          }
        }
        n2956 = case shown="True" "OPEN 2" {
          frame False {
          }
          frame True {
            (unwired) 0  # existing file
            w3840 = "Choose a datalog file to open"  # prompt
            n2957 = local write "OPEN 2"(FALSE ("OPEN 1")) -> ()
            n2958 = String To Path(string="C:\\LAB-IQ\\Data\\") -> (path=w3825:path)
            n2959 = File Dialog(6:"*.dgf" ("pattern"), 7:w3840, 11:w3825) -> (0:w3823:errorcluster, 3:w3831:path)  [unwired: 4 in, 2 out]
            n2960 = Unbundle(w3823) -> ()  [unwired: 3 out]
            n2961 = Strip Path(path=w3831) -> (name=w3829:string)  [unwired: 1 out]
            n2962 = Path To String(path=w3831) -> (string=w3826:string)
            "string1 2" <- w3826
            n2963 = Match Pattern(string=w3829, regular expression=".dgf") -> (before substring=→"String Control 3":string)  [unwired: 1 in, 3 out]
            n2964 = Match Pattern(string=w3826, regular expression=".dgf" ("substring (\"\")")) -> (before substring=w3837:string)  [unwired: 1 in, 3 out]
            n2965 = Concatenate Strings(w3837, ".duf" ("Substring")) -> (w3834:string)
            n2966 = String To Path(string=w3834) -> (path=w3832:path)
